vi "Update.vi"(8 "error in (no error)":errorcluster, 10 "Controls":T1, 11 "Cheat in":refnum<class "Cheat.lvclass">) -> (0 "error out":errorcluster, 3 "Cheat out":refnum<class "Cheat.lvclass">)   [LabVIEW 2019, in "RT_Game.lvlib" / "Cheat.lvclass"]
uses:
  Cheat.lvclass
  Engine/Controls.ctl
  Engine/ControlPlayer.ctl
  Cheat.lvclass/Cheat.ctl
  CheatControl.ctl
  Engine/Globals.vi
  Engine/Engine.lvclass
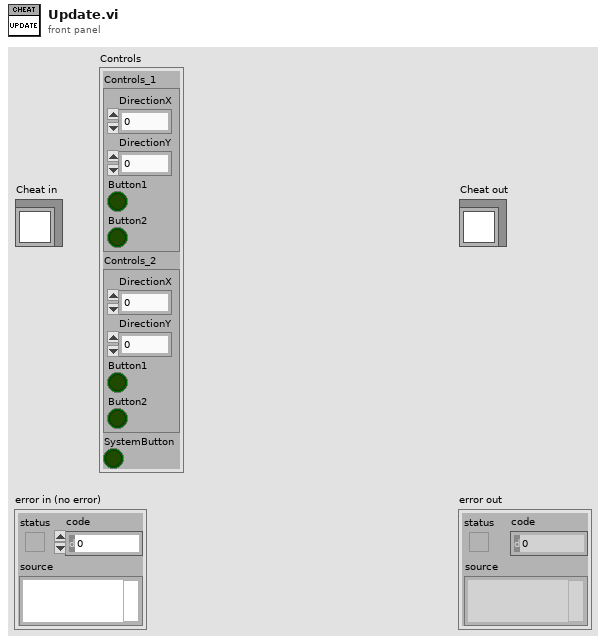
[diagram p1: front panel]
types:
  T1 = typedef "RT_Game.lvlib/Engine.lvclass/Controls.ctl" = cluster{"Controls_1":T2, "Controls_2":cluster{"DirectionX":i8, "DirectionY":i8, "Button1":bool, "Button2":bool}, "SystemButton":bool}
  T2 = typedef "RT_Game.lvlib/Engine.lvclass/ControlPlayer.ctl" = cluster{"DirectionX":i8, "DirectionY":i8, "Button1":bool, "Button2":bool}
  T3 = typedef "RT_Game.lvlib/Cheat.lvclass/CheatControl.ctl" = enum16{"none", "left1", "left2", "right1", "right2", "leftStick", "rightStick"}
  T4 = cluster{"DirectionX":i8, "DirectionY":i8, "Button1":bool, "Button2":bool}
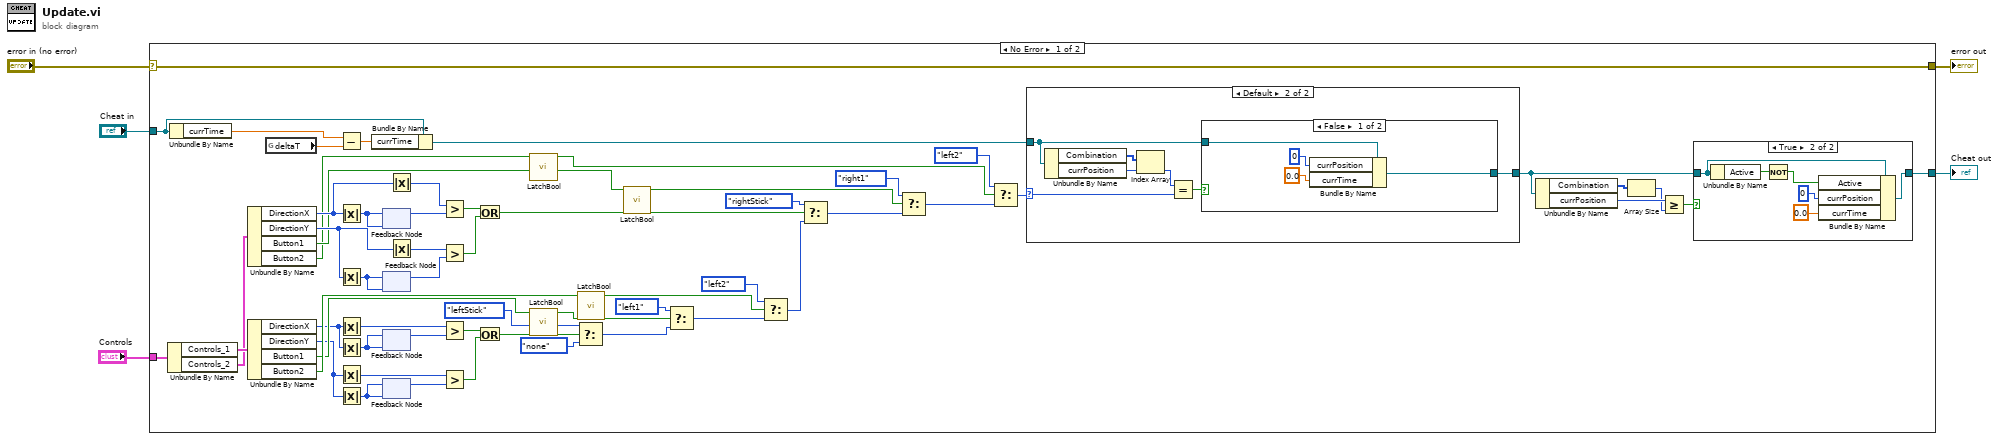
[diagram p0: block diagram]
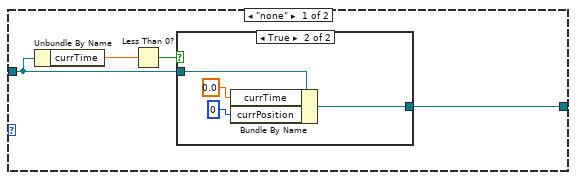
[diagram p2: hidden frame]
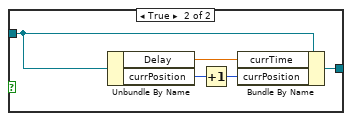
[diagram p4: hidden frame]
diagram:
  n1 = case shown="No Error" "error in (no error)" {
    selector: "error in (no error)" -> [w63 w97]
    tunnel: [w63 w97] -> w4
    tunnel: [w11 w96] -> w2
    tunnel: "Cheat in" -> [w16 w96]
    tunnel: "Controls" -> [w62 _]
    frame No Error {
      n2 = Unbundle By Name(w62) -> ("Controls_1"=w61:T2, "Controls_2"=w40:T4)
      n3 = Unbundle By Name(w16) -> ("currTime"=w15:dbl)
      n4 = Unbundle By Name(w40) -> ("DirectionX"=w43:i8, "DirectionY"=w50:i8, "Button1"=w42:bool, "Button2"=w41:bool)
      n5 = Unbundle By Name(w61) -> ("DirectionX"=w58:i8, "DirectionY"=w51:i8, "Button1"=w59:bool, "Button2"=w60:bool)
      n6 = global read "Globals.vi" "deltaT"() -> (w13:dbl)
      n7 = Subtract(x=w15, y=w13) -> (x-y=w14:dbl)
      n8 = Absolute Value(x=w43) -> (abs(x)=w44:i8)
      n9 = Absolute Value(x=w50) -> (abs(x)=w49:i8)
      n10 = Absolute Value(x=w58) -> (abs(x)=w56:i8)
      n11 = Absolute Value(x=w58) -> (abs(x)=w57:i8)
      n12 = Absolute Value(x=w51) -> (abs(x)=w53:i8)
      n13 = Absolute Value(x=w51) -> (abs(x)=w52:i8)
      n14 = Bundle By Name(cluster=w16, "currTime"=w14) -> (w12:refnum<class "Cheat.lvclass">)
      n15 = feedback #1(w44) -> (w46:i8)
      n16 = feedback-in #1(w44) -> ()
      n17 = feedback #2(w49) -> (w47:i8)
      n18 = feedback-in #2(w49) -> ()
      n19 = feedback-in #3(w57) -> ()
      n20 = feedback #3(w57) -> (w55:i8)
      n21 = feedback #4(w52) -> (w54:i8)
      n22 = feedback-in #4(w52) -> ()
      n23 = Absolute Value(x=w43) -> (abs(x)=w45:i8)
      n24 = Absolute Value(x=w50) -> (abs(x)=w48:i8)
      n25 = Greater?(x=w45, y=w46) -> (0:w37:bool)
      n26 = Greater?(x=w48, y=w47) -> (0:w36:bool)
      n27 = Greater?(x=w56, y=w55) -> (0:w39:bool)
      n28 = Greater?(x=w53, y=w54) -> (0:w38:bool)
      n29 = Or(x=w37, y=w36) -> (x .or. y?=w29:bool)
      n30 = Or(x=w39, y=w38) -> (x .or. y?=w35:bool)
      n31 = call "LatchBool.vi"("Boolean"=w41) -> ("Latched Boolean"=w25:bool)  [unwired: 10 in]
      n32 = call "LatchBool.vi"("Boolean"=w59) -> ("Latched Boolean"=w33:bool)  [unwired: 10 in]
      n33 = Select(t=CheatControl."leftStick" ("controls"), s=w35, f=CheatControl."none") -> (s? t:f=w34:T3)
      n34 = call "LatchBool.vi"("Boolean"=w60) -> ("Latched Boolean"=w31:bool)  [unwired: 10 in]
      n35 = call "LatchBool.vi"("Boolean"=w42) -> ("Latched Boolean"=w27:bool)  [unwired: 10 in]
      n36 = Select(t=CheatControl."left1", s=w33, f=w34) -> (s? t:f=w32:T3)
      n37 = Select(t=CheatControl."left2", s=w31, f=w32) -> (s? t:f=w30:T3)
      n38 = Select(t=CheatControl."rightStick", s=w29, f=w30) -> (s? t:f=w28:T3)
      n39 = Select(t=CheatControl."right1", s=w27, f=w28) -> (s? t:f=w26:T3)
      n40 = Select(t=CheatControl."left2", s=w25, f=w26) -> (s? t:f=w17:T3)
      n41 = case shown="Default" w17 {
        selector: w17 -> [_ w76]
        tunnel: [w66 w75] -> w7
        tunnel: w12 -> [w67 w74]
        frame "none" {
          n42 = Unbundle By Name(w67) -> ("currTime"=w65:dbl)
          n43 = Less Than 0?(x=w65) -> (x < 0?=w64:bool)
          n44 = case shown="True" w64 {
            tunnel: w67 -> [w68 w72]
            tunnel: [w68 w71] -> w66
            frame False {
            }
            frame True {
              n45 = Bundle By Name(cluster=w72, "currTime"=0.0, "currPosition"=i16 0) -> (w71:refnum<class "Cheat.lvclass">)
            }
          }
        }
        frame Default {
          n46 = Unbundle By Name(w74) -> ("Combination"=w79:T3[], "currPosition"=w78:i16)
          n47 = Index Array(array=w79, index=w78) -> (element=w77:T3)
          n48 = Equal?(x=w77, y=w76) -> (x = y?=w73:bool)
          n49 = case shown="False" w73 {
            tunnel: [w82 w88] -> w75
            tunnel: w74 -> [w83 w84]
            frame False {
              n50 = Bundle By Name(cluster=w83, "currPosition"=i16 0, "currTime"=0.0) -> (w82:refnum<class "Cheat.lvclass">)
            }
            frame True {
              n51 = Unbundle By Name(w84) -> ("Delay"=w87:dbl, "currPosition"=w86:i16)
              n52 = Increment(x=w86) -> (x+1=w85:i16)
              n53 = Bundle By Name(cluster=w84, "currTime"=w87, "currPosition"=w85) -> (w88:refnum<class "Cheat.lvclass">)
            }
          }
        }
      }
      n54 = Unbundle By Name(w7) -> ("Combination"=w10:T3[], "currPosition"=w9:i16)
      n55 = Array Size(array=w10) -> (size(s)=w8:i32)
      n56 = Greater Or Equal?(x=w9, y=w8) -> (x >= y?=w6:bool)
      n57 = case shown="True" w6 {
        tunnel: [w89 w95] -> w11
        tunnel: w7 -> [w89 w94]
        frame False {
        }
        frame True {
          n58 = Unbundle By Name(w94) -> ("Active"=w93:bool)
          n59 = Not(x=w93) -> (.not. x?=w92:bool)
          n60 = Bundle By Name(cluster=w94, "Active"=w92, "currPosition"=i16 0, "currTime"=0.0) -> (w95:refnum<class "Cheat.lvclass">)
        }
      }
    }
    frame Error {
    }
  }
  "error out" <- w4
  "Cheat out" <- w2
